vi "New Heartbeat Message.vi"() -> (0 "Heartbeat Message":cluster{"Type":string, "Message":string})   [LabVIEW 2016]
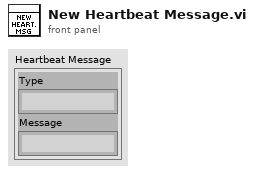
[diagram p1: front panel]
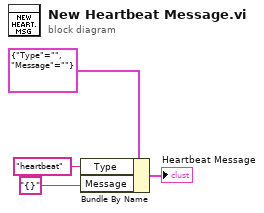
[diagram p0: block diagram]
diagram:
  n1 = Bundle By Name(cluster=cluster{"Type":string, "Message":string} {"Type"="", "Message"=""}, "Type"="heartbeat", "Message"="{}") -> (→"Heartbeat Message":cluster{"Type":string, "Message":string})
